vi "Register UI user events.vi"(8 "error in (no error)":errorcluster, 11 "Execution UI In":refnum<class "Execution UI.lvclass">) -> (0 "error out":errorcluster, 2 "Event Registration Refnum":refnum<event-registration>, 3 "Execution UI Out":refnum<class "Execution UI.lvclass">)   [LabVIEW 2020, in "Execution UI.lvclass"]
uses:
  Execution UI.lvclass
  Execution UI.lvclass/Execution UI.ctl
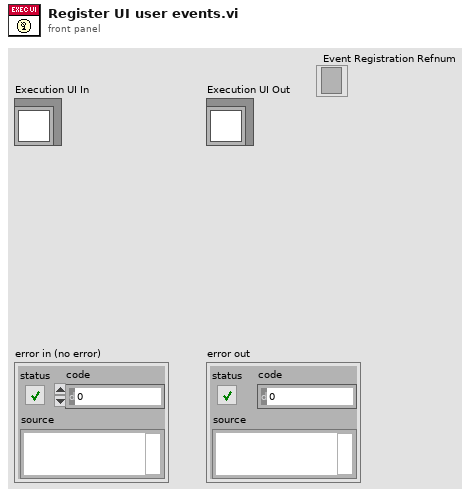
[diagram p1: front panel]
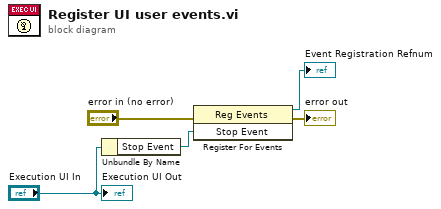
[diagram p0: block diagram]
diagram:
  n1 = Unbundle By Name("Execution UI In") -> ("Stop Event"=w1:refnum<user-event>)
  n2 = register-events(error in="error in (no error)", w1) -> (reference out=→"Event Registration Refnum":refnum<event-registration>, error out=→"error out":errorcluster)  [unwired: 1 in]
  "Execution UI Out" <- "Execution UI In"
